vi "Outline cyc Time.vi"(0 "Online_Table":T1) -> (1 "Pstates":bool, 6 "Repair":i32)   [LabVIEW 2014]
uses:
  Type'def/Online_Table.ctl
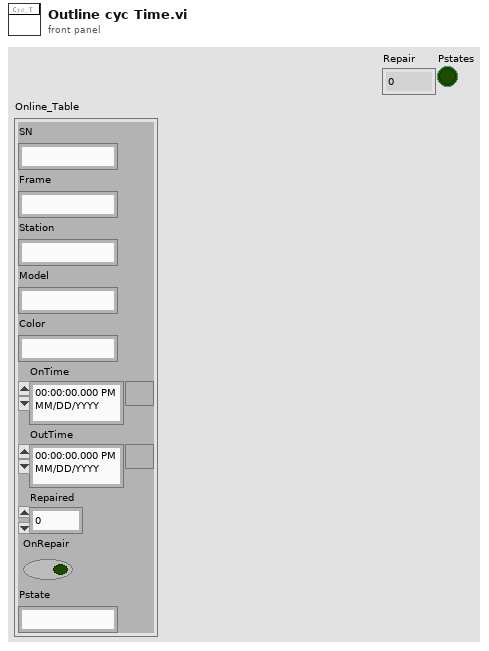
[diagram p1: front panel]
types:
  T1 = typedef "Online_Table.ctl" = cluster{"SN":string, "Frame":string, "Station":string, "Model":string, "Color":string, "OnTime":timestamp, "OutTime":timestamp, "Repaired":i32, "OnRepair":bool, "Pstate":string}
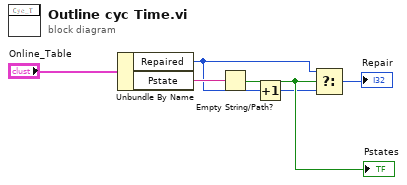
[diagram p0: block diagram]
diagram:
  n1 = Unbundle By Name("Online_Table") -> ("Repaired"=w2:i32, "Pstate"=w6:string)
  n2 = Empty String/Path?(string/path=w6) -> (empty?=w4:bool)
  "Pstates" <- w4
  n3 = Increment(x=w2) -> (x+1=w3:i32)
  n4 = Select(t=w2, s=w4, f=w3) -> (s? t:f=→"Repair":i32)
